vi "Generate_path.vi"(11 "name or relative path":string) -> (2 "MyFile":path)   [LabVIEW 2018]
doc: "Realtive path"
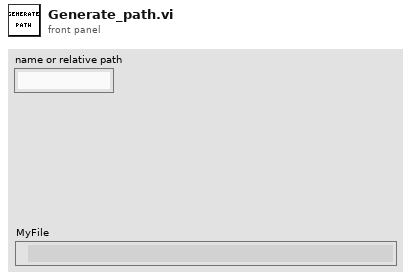
[diagram p1: front panel]
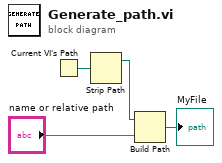
[diagram p0: block diagram]
diagram:
  n1 = Current VI's Path() -> (path=w2:path)
  n2 = Strip Path(path=w2) -> (stripped path=w3:path)  [unwired: 1 out]
  n3 = Build Path(base path=w3, name or relative path="name or relative path") -> (appended path=→"MyFile":path)
